vi "ZStack.vi"(0 "object in":refnum<class "Application.lvclass">, 1 "Top":dbl, 2 "Bottom":dbl, 4 "Step Size":dbl, 5 "error in (no error)":errorcluster) -> (14 "object out":refnum<class "Application.lvclass">, 19 "error out":errorcluster)   [LabVIEW 2021, in "Application.lvclass"]
uses:
  Application.lvclass
  Prior_Zmotor_class/Prior_Zmotor.lvclass
  Hamamatsu_class/Hamamatsu.lvclass
  Application.lvclass/Application.ctl
panel:
  out "Position (um) 2":dbl
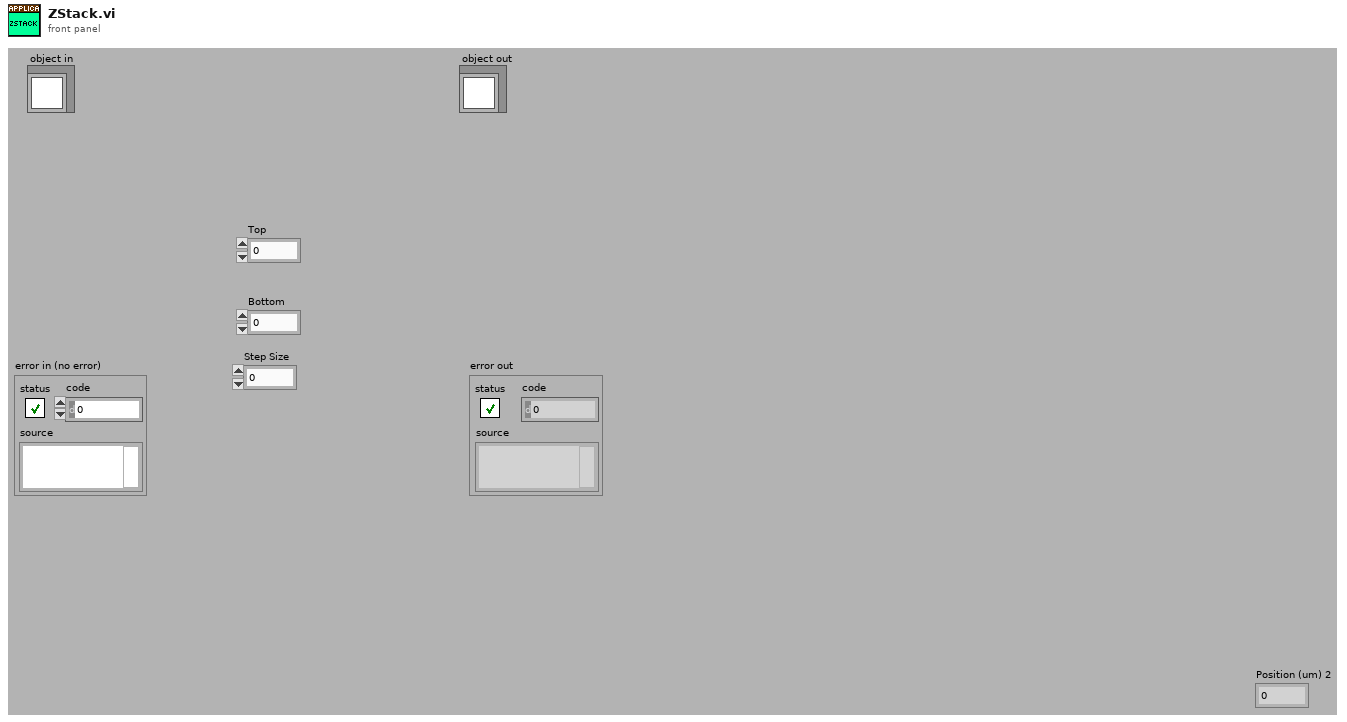
[diagram p1: front panel]
types:
  T1 = enum16{"open", "open or create", "create or replace", "create", "open (read-only)"}
  T2 = typedef "IMAQ Image.ctl" = refnum<image>
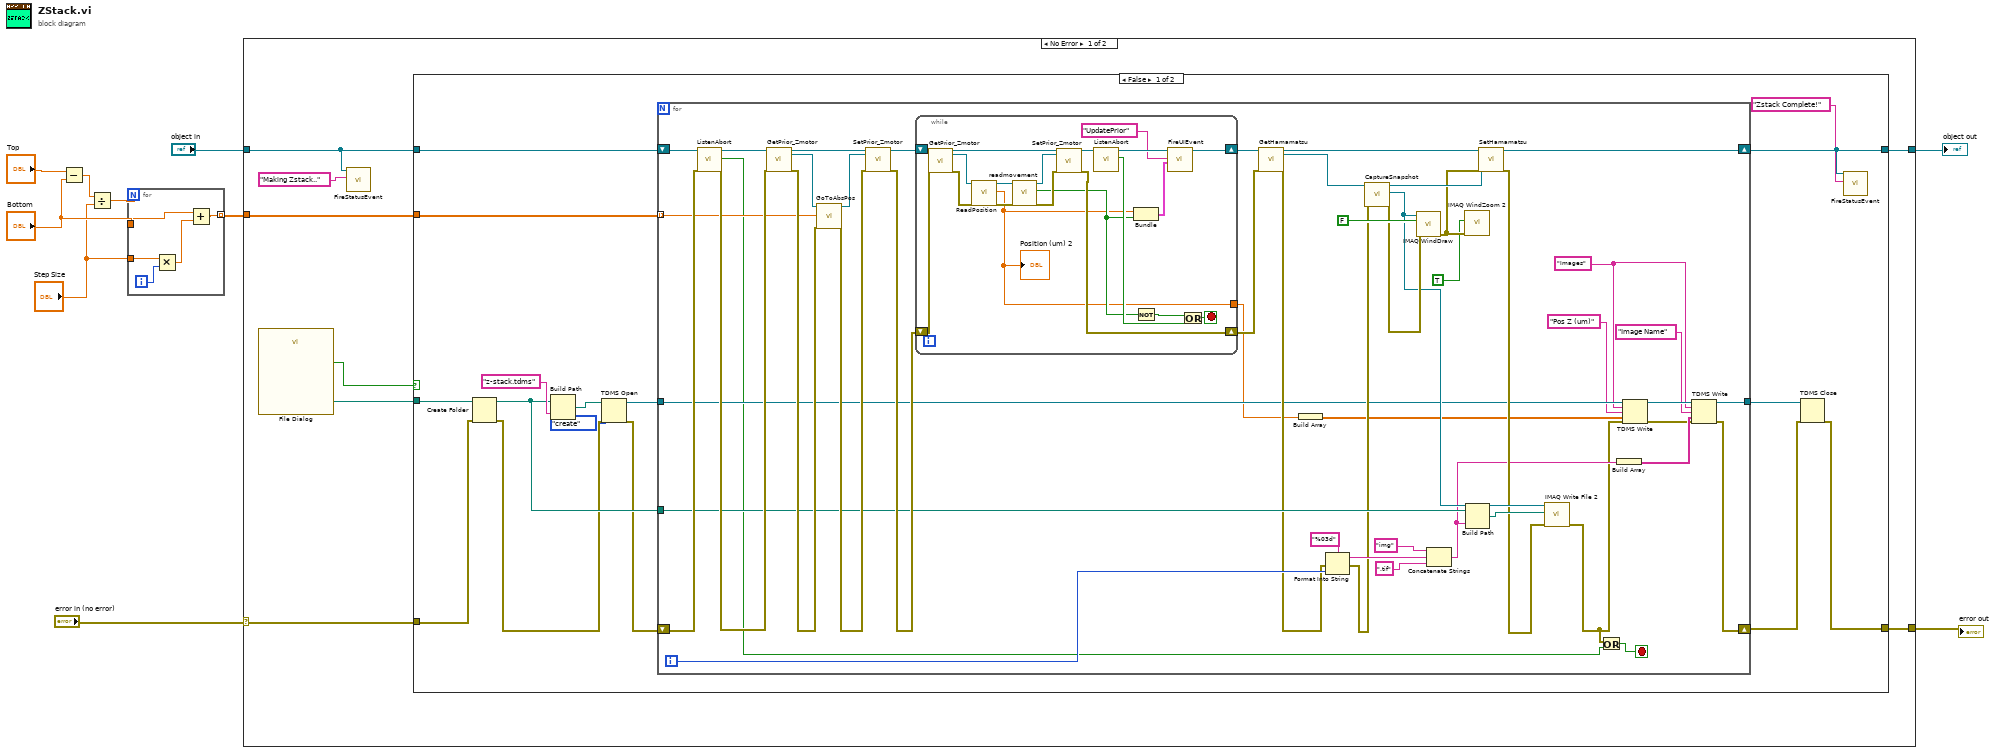
[diagram p0: block diagram]
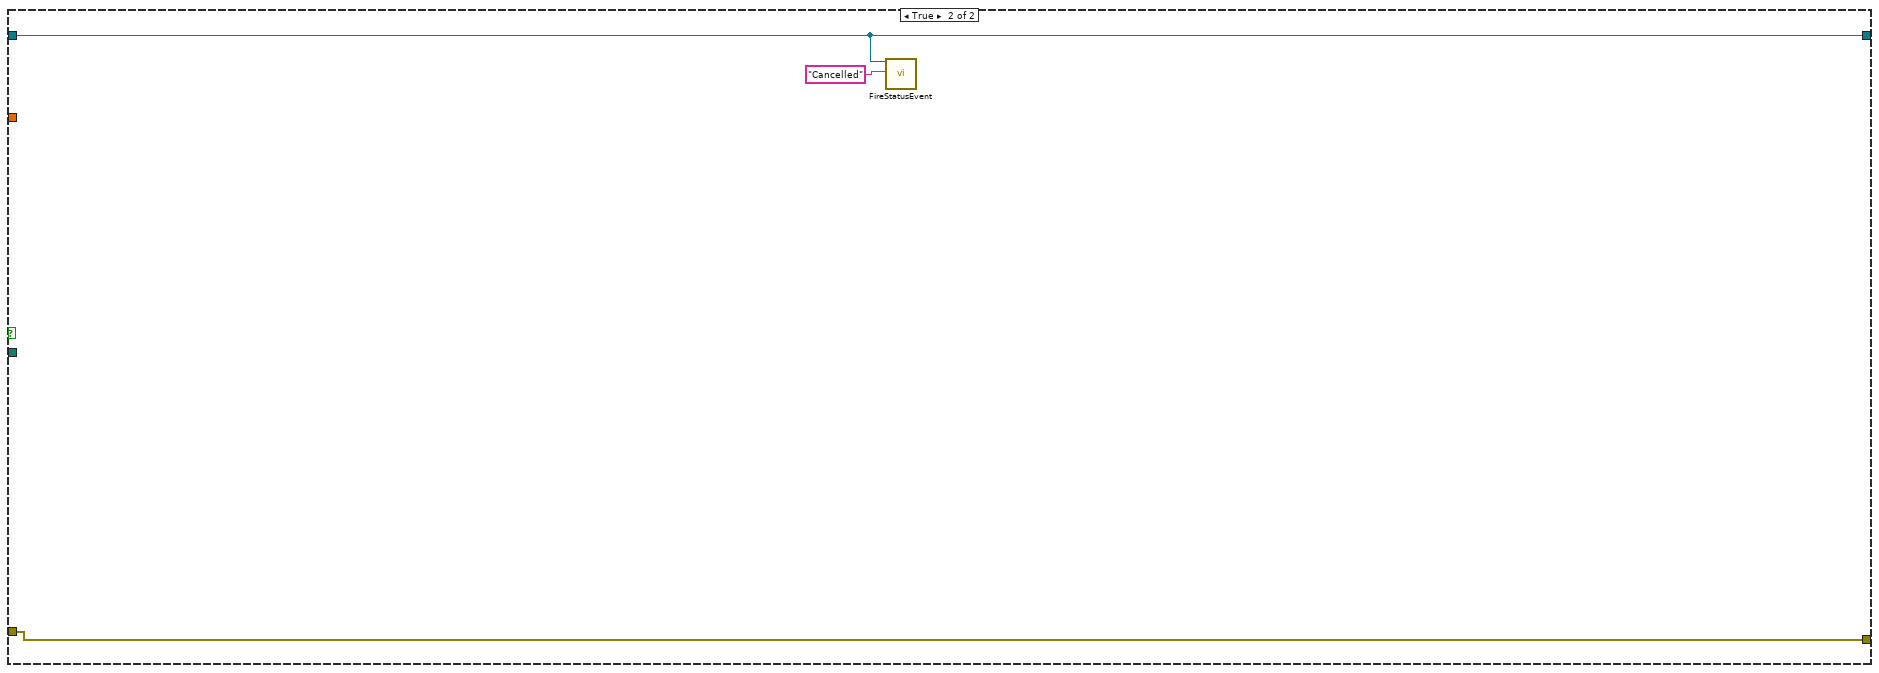
[diagram p2: hidden frame]
diagram:
  n1 = Subtract(x="Top", y="Bottom") -> (x-y=w5:dbl)
  n2 = Divide(x=w5, y="Step Size") -> (x/y=w4:dbl)
  n3 = for {
    N: w4 -> [_]
    tunnel: "Bottom" -> [w12]
    tunnel: "Step Size" -> [w14]
    tunnel: [w11] -> w1 mode=indexing
    i -> [w15]
    n4 = Multiply(x=w14, y=w15) -> (x*y=w13:dbl)
    n5 = Add(x=w12, y=w13) -> (x+y=w11:dbl)
  }
  n6 = case shown="No Error" "error in (no error)" {
    selector: "error in (no error)" -> [w18 w112]
    tunnel: [w23 w112] -> w9
    tunnel: [w19 w111] -> w7
    tunnel: "object in" -> [w21 w111]
    tunnel: w1 -> [w22 _]
    frame No Error {
      n7 = call "File Dialog"() -> ("selected path"=w17:path, "cancelled"=w16:bool)  [unwired: 12 in, 2 out]
      n8 = call-dynamic "FireStatusEvent.vi"("object in"=w21, "Status"="Making Zstack..") -> ()  [unwired: 16 in, 2 out]
      n9 = case shown="False" w16 {
        tunnel: [w25 w108] -> w23
        tunnel: w22 -> [w39 _]
        tunnel: w21 -> [w38 w109]
        tunnel: [w37 w109] -> w19
        tunnel: w18 -> [w35 w108]
        tunnel: w17 -> [w34 _]
        frame False {
          n10 = Create Folder(path (use dialog)=w34, error in=w35) -> (created path=w31:path, error out=w29:errorcluster)  [unwired: 1 in, 1 out]
          n11 = Build Path(base path=w31, name or relative path="z-stack.tdms") -> (appended path=w33:path)
          n12 = TDMS Open(8:w29, 10:T1."create" ("operation (0:open)"), 11:w33) -> (0:w28:errorcluster, 3:w30:refnum<k34>)  [unwired: 4 in]
          n13 = for {
            shift-right: [w78] -> w37
            shift-left: w38 -> [w77]
            shift-right: [w41] -> w26
            shift-left: w28 -> [w76]
            tunnel: w39 -> [w66] mode=indexing
            tunnel: w31 -> [w58]
            tunnel: w30 -> [w54]
            tunnel: [w40] -> w27
            i -> [w59]
            stop <- w52 stop-if-true
            w47 = "Images"
            n14 = call-dynamic "ListenAbort.vi"("object in"=w77, "error in (no error)"=w76) -> ("object out"=w74:refnum<class "Application.lvclass">, "Abort?"=w53:bool, "error out"=w72:errorcluster)  [unwired: 15 in]
            n15 = call-dynamic "GetPrior_Zmotor.vi"("object in"=w74, "error in (no error)"=w72) -> ("object out"=w73:refnum<class "Application.lvclass">, "Prior_Zmotor"=w70:refnum<class "Prior_Zmotor.lvclass">, "error out"=w69:errorcluster)  [unwired: 15 in]
            n16 = call-dynamic "GoToAbsPos.vi"("object in"=w70, "Pos (um)"=w66, "error in (no error)"=w69) -> ("object out"=w67:refnum<class "Prior_Zmotor.lvclass">, "error out"=w68:errorcluster)  [unwired: 14 in, 1 out]
            n17 = call-dynamic "SetPrior_Zmotor.vi"("object in"=w73, "Prior_Zmotor"=w67, "error in (no error)"=w68) -> ("object out"=w75:refnum<class "Application.lvclass">, "error out"=w71:errorcluster)  [unwired: 15 in]
            n18 = while {
              shift-right: [w92] -> w80
              shift-left: w75 -> [w103]
              shift-right: [w99] -> w79
              shift-left: w71 -> [w102]
              tunnel: [w88] -> w51
              stop <- w93 stop-if-true
              n19 = call-dynamic "GetPrior_Zmotor.vi"("object in"=w103, "error in (no error)"=w102) -> ("object out"=w107:refnum<class "Application.lvclass">, "Prior_Zmotor"=w106:refnum<class "Prior_Zmotor.lvclass">, "error out"=w104:errorcluster)  [unwired: 15 in]
              n20 = call-dynamic "ReadPosition.vi"("object in"=w106, "error in (no error)"=w104) -> ("object out"=w105:refnum<class "Prior_Zmotor.lvclass">, "Position (um)"=w88:dbl, "error out"=w100:errorcluster)  [unwired: 15 in]
              "Position (um) 2" <- w88
              n21 = call-dynamic "readmovement.vi"("object in"=w105, "error in (no error)"=w100) -> ("object out"=w101:refnum<class "Prior_Zmotor.lvclass">, "IsMoving?"=w90:bool, "error out"=w98:errorcluster)  [unwired: 15 in]
              n22 = call-dynamic "SetPrior_Zmotor.vi"("object in"=w107, "Prior_Zmotor"=w101, "error in (no error)"=w98) -> ("object out"=w97:refnum<class "Application.lvclass">, "error out"=w99:errorcluster)  [unwired: 15 in]
              n23 = call-dynamic "ListenAbort.vi"("object in"=w97) -> ("object out"=w96:refnum<class "Application.lvclass">, "Abort?"=w94:bool)  [unwired: 16 in, 1 out]
              n24 = Bundle("Position (um)"=w88, "IsMoving?"=w90) -> (w89:cluster{"Position (um)":dbl, "IsMoving?":bool})  [unwired: 1 in]
              n25 = Not(x=w90) -> (.not. x?=w95:bool)
              n26 = call-dynamic "FireUIEvent.vi"("object in"=w96, "Message"="UpdatePrior", "Message Data"=w89) -> ("object out"=w92:refnum<class "Application.lvclass">)  [unwired: 15 in, 1 out]
              n27 = Or(x=w95, y=w94) -> (x .or. y?=w93:bool)
            }
            n28 = call-dynamic "GetHamamatsu.vi"("object in"=w80, "error in (no error)"=w79) -> ("object out"=w87:refnum<class "Application.lvclass">, "Hamamatsu"=w86:refnum<class "Hamamatsu.lvclass">, "error out"=w57:errorcluster)  [unwired: 15 in]
            n29 = Build Array(w51) -> (w50:dbl[])
            n30 = Format Into String(format string="%03d", error in=w57, w59) -> (resulting string=w63:string, error out=w56:errorcluster)  [unwired: 1 in]
            n31 = call-dynamic "CaptureSnapshot.vi"("object in"=w86, "error in (no error)"=w56) -> ("object out"=w85:refnum<class "Hamamatsu.lvclass">, "FreeRunningImage"=w60:T2, "error out"=w81:errorcluster)  [unwired: 14 in, 1 out]
            n32 = call "IMAQ WindDraw"("Resize to Image Size? (Y)"=FALSE, "error in (no error)"=w81, "Image"=w60) -> ("error out"=w83:errorcluster)  [unwired: 7 in, 1 out]
            n33 = Concatenate Strings("img" ("string"), w63, ".tif" ("string")) -> (w45:string)
            n34 = call "IMAQ WindZoom 2"("error in (no error)"=w83, "Zoom to Fit? (False)"=TRUE) -> ()  [unwired: 6 in, 4 out]
            n35 = Build Path(base path=w58, name or relative path=w45) -> (appended path=w62:path)
            n36 = call-dynamic "SetHamamatsu.vi"("object in"=w87, "Hamamatsu"=w85, "error in (no error)"=w83) -> ("object out"=w78:refnum<class "Application.lvclass">, "error out"=w55:errorcluster)  [unwired: 15 in]
            n37 = call-poly "IMAQ Write File 2"("error in (no error)"=w55, "File Path"=w62, "Image"=w60) -> ("error out"=w42:errorcluster)  [unwired: 7 in, 1 out]
            n38 = Or(x=w42, y=w53) -> (x .or. y?=w52:bool)
            n39 = Build Array(w45) -> (w44:string[])
            n40 = TDMS Write(0:w54, 5:w47, 7:"Pos Z (um)", 9:w50, 11:w42) -> (4:w48:refnum<k34>, 15:w43:errorcluster)  [unwired: 1 in, 2 out]
            n41 = TDMS Write(0:w48, 5:w47, 7:"Image Name", 9:w44, 11:w43) -> (4:w40:refnum<k34>, 15:w41:errorcluster)  [unwired: 1 in, 2 out]
          }
          n42 = TDMS Close(8:w26, 11:w27) -> (0:w25:errorcluster)  [unwired: 1 out]
          n43 = call-dynamic "FireStatusEvent.vi"("object in"=w37, "Status"="Zstack Complete!") -> ()  [unwired: 16 in, 2 out]
        }
        frame True {
          n44 = call-dynamic "FireStatusEvent.vi"("object in"=w109, "Status"="Cancelled") -> ()  [unwired: 16 in, 2 out]
        }
      }
    }
    frame Error {
    }
  }
  "error out" <- w9
  "object out" <- w7
